vi "CANOpen Addon GUID Lookup Global.vi"() -> ()   [LabVIEW 2021, in "CANOpen Addon Shared.lvlib"]
doc: "Use this Global VI to access the GUIDs assigned to the page resources of the Custom Device."
uses:
  CANOpen Addon Shared.lvlib
panel:
  in  "Tab Control":enum32{"CD", "PDO", "SDO", "NMT"}(tab)
  in  "CANOpen RPDO Channel GUID":string="DE69C061-F71C-4601-910F-EC06EE56C86C"
  in  "Prop_Bus Setting Scan and print":string="Scan and print"
  in  "CANOpen Engine Missed":string="Late counts"
  in  "CANOpen Engine Iteration":string="Iteration duration"
  in  "CANOpen Engine Status":string="Status"
  in  "Prop_Bus Setting Sync Enabled":string="Enable SYNC"
  in  "Custom Device GUID":string="ee2eec27-2ab7-4da4-b26b-0d826264739c"
  in  "CANOpen Device Node GUID":string="30ee7416-8e02-4aa2-8b9c-c256d8ed97d5"
  in  "CANOpen Device Node Name":string="Device Node"
  in  "Custom Device Disabled GUID":string="b0754a10-6e57-4997-b995-895c0828dacd"
  in  "Prop_Bus Settings":string="CANOpen Bus Settings"
  in  "Prop_Bus Setting Baud Rate":string="Baud Rate"
  in  "Prop_Bus Setting Termination":string="Termination"
  in  "Prop_Bus Setting Sync Period":string="Sync Period (ms)"
  in  "Prop_Bus Setting Interface":string="CANOpen Interface Name"
  in  "CANOpen Command Reset Bus":string="Reset Bus"
  in  "CANOpen Bus Command GUID":string="d746360c-3e97-4e77-b411-872b8f57c1d4"
  in  "CANOpen Bus Command Name":string="CANopen Engine"
  in  "Prop_Bus Setting Enable 9881":string="Enable 9881"
  in  "Prop_Bus Setting RIO Device":string="RIO Device"
  in  "CANOpen Add Node GUID":string="33398edb-ff6b-43ad-b42c-50e0a0d68fac"
  in  "CANOpen Duplicate Node GUID":string="c1cabacc-3d01-49d5-b055-4ef04d206838"
  in  "CANOpen Refresh Node GUID":string="870003e8-09bd-4a3b-a7ca-f5c9f1d16aa4"
  in  "CANOpen TPDO Channel GUID":string="29165bcc-5b74-4ff4-a426-96512b74f616"
  in  "Prop_9881 Bitfile":string="9881 Bitfile"
  in  "Prop_PDO Parameter Name":string="Parameter Name"
  in  "CANOpen RPDOs GUID":string="a6766e6a-de04-4fdb-a423-a2081741c0e8"
  in  "CANOpen TPDOs GUID":string="058a6a92-3f0d-49e3-a3a0-9535fbe5a49e"
  in  "CANOpen RPDOs Name":string="RPDOs"
  in  "CANOpen TPDOs Name":string="TPDOs"
  in  "CANOpen Add RPDO GUID":string="28e29660-92b3-44b9-a0a1-97cd359da2d3"
  in  "CANOpen Add TPDO GUID":string="5546cecb-dffa-420d-be45-0b533e545aa0"
  in  "CANOpen PDO GUID":string="0e998ef5-190c-48b6-92bd-d5f6d14f96b8"
  in  "Prop_PDO Channel":string="PDO Channel"
  in  "Prop_PDO Settings":string="PDO Settings"
  in  "Prop_PDO Parameter Scale Factor":string="Scale Factor"
  in  "Prop_PDO Parameter Scale Offset":string="Scale Offset"
  in  "Prop_PDO Parameter Byte Offset":string="Byte Offset"
  in  "Prop_PDO Parameter Bit Offset":string="Bit Offset"
  in  "Prop_PDO Parameter Data Type":string="Data Type"
  in  "Prop_PDO Parameter Settings":string="PDO Parameter Settings"
  in  "Prop_PDO Parameter Byte Order":string="Byte Order"
  in  "CANOpen Dynamic SDOs Write Req Section GUID":string="3097BF4C-8B3B-4279-9609-A1E06BBA9A61"
  in  "CANOpen Dynamic SDOs Write Resp Section GUID":string="B538C8C3-1320-40E6-85C4-5CBF861E5FF7"
  in  "CANOpen Dynamic SDOs Read Req Section GUID":string="84B55C87-CCAB-4A59-989A-F3927336083A"
  in  "CANOpen Dynamic SDOs Read Resp Section GUID":string="11BBA49E-62B9-4BE5-94B9-DFD78A3C50D4"
  in  "CANOpen SDOs - Dynamic Subsection GUID":string="C0059D1D-3ED5-454F-9A27-1F2434054ECF"
  in  "CANOpen Resp List SDOs Name":string="Status of List SDO"
  in  "CANOpen Dynamic SDOs section Name":string="SDOs - Dynamic"
  in  "CANOpen SDOs - Dynamic GUID":string="498D62A3-F405-4B08-B47B-C5A393B4DBAF"
  in  "Prop_SDO Settings - Dynamic":string="SDO Settings - dynamic"
  in  "CANOpen SDOs - Startup GUID":string="4ac413d5-b28b-4132-8469-846c133003cb"
  in  "CANOpen SDOs Name":string="SDOs - Startup"
  in  "CANOpen SDO GUID":string="ea1c03c6-7bc5-4a9b-b7be-6b905fdf2687"
  in  "CANOpen SDOs - List GUID":string="4009128c-3f61-49ec-a349-cb63a112dd75"
  in  "Prop_SDO Settings - list dynamic":string="SDO Settings - list dynamic"
  in  "CANOpen SDOs main name":string="SDOs"
  in  "CANOpen Receive Status GUID":string="B4588A11-20C8-4448-980C-55D7BC0F1605"
  in  "CANOpen List SDOs section Name":string="SDOs - List"
  in  "CANOpen Send List SDOs Name":string="Send specific list SDO"
  in  "Prop_SDO Settings":string="SDO Settings"
  in  "CANOpen Add SDOs GUID":string="ba5535c9-1052-42b9-a99b-a7a4548c3bfe"
  in  "CANOpen Edit SDOs GUID":string="1cf17f76-dd6b-43a3-9629-5f3997969536"
  in  "CANOpen SDOs main GUID":string="b40cd152-95d7-469e-822f-e3172d1a480a"
  in  "CANOpen List SDOs Req GUID":string="aab1a3c1-d588-4927-aa76-77b77a44aad7"
  in  "CANOpen Dynamic SDOs Write Req GUID":string="51538351-12DA-4E79-8082-0EFA430E7DD8"
  in  "CANOpen Dynamic SDOs Write Resp GUID":string="4F260029-3D47-4DD5-AC89-DDD2EA29783B"
  in  "CANOpen Dynamic SDOs Read Req GUID":string="96EBA813-65BB-4356-9ACB-EB1E8C7D1BA9"
  in  "CANOpen Dynamic SDOs Read Resp GUID":string="4437B1E7-4881-413A-A86D-C6CCD713B80B"
  in  "CANOpen List SDOs Resp GUID":string="2CA7D733-94A4-4949-AD76-6DC6B0B520E8"
  in  "Prop_NMT Node init static SDO state":string="Node init static SDO state"
  in  "Prop_NMT Node run state":string="Node run state"
  in  "Prop_NMT Delay for opp. state (ms)":string="Delay for opp. state (ms)"
  in  "Prop_NMT HB NG":string="HB NG"
  in  "Prop_NMT Stop and Reset on Shutdown":string="Stop and Reset on Shutdown"
  in  "Prop_NMT Emergency":string="Emergency"
  in  "CANOpen NMTs GUID":string="E973F48E-341C-44BD-96D0-0955FA5D4E9C"
  in  "CANOpen NMTs main name":string="NMTs"
  in  "CANOpen Send NMT GUID":string="1344E165-397F-4945-9CF4-5D878AFF51A5"
  in  "CANOpen Send NMT Name":string="NMT command"
  in  "Prop_NMT Settings":string="Prop_NMT Settings"
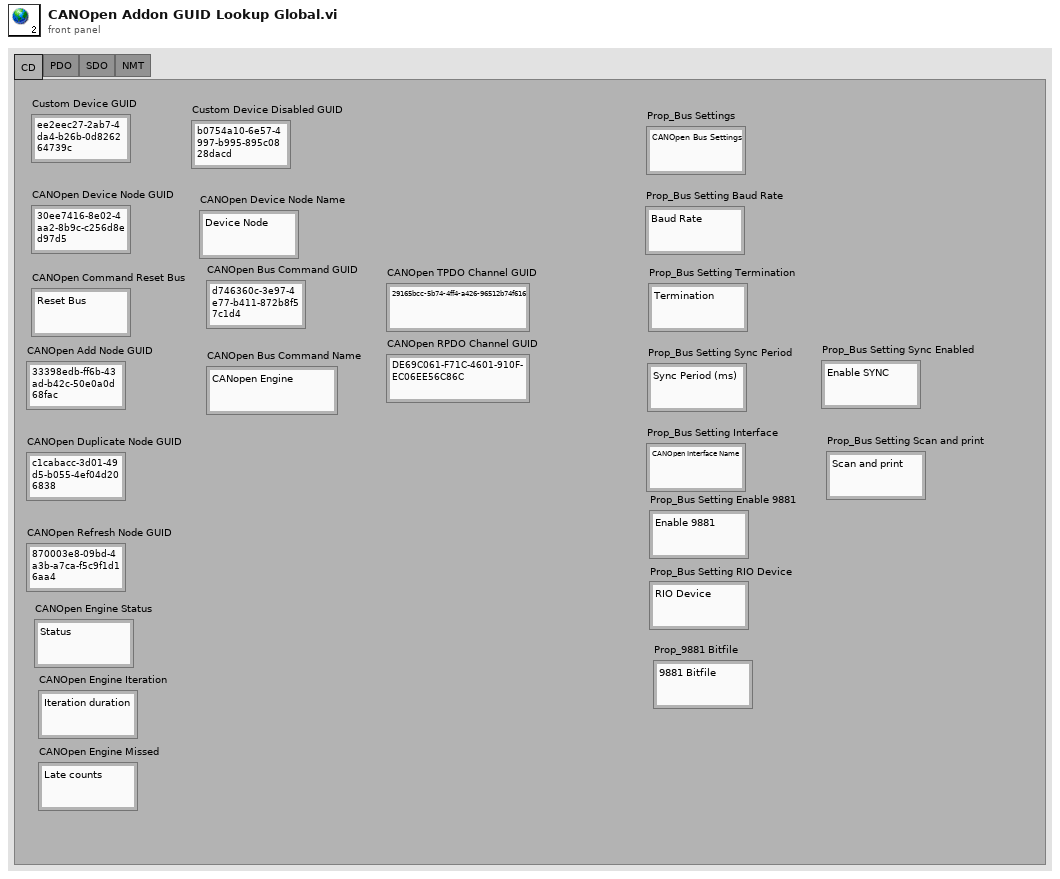
[diagram p1: front panel]
diagram:
